vi "test27-MappingRelationshipByLocalRegistration_WithoutSubcriberName.vi"(8 "error in (no error)":errorcluster, 11 "TestCase in":refnum<class "testcase-CSMBroadcast.lvclass">) -> (0 "error out":errorcluster, 3 "TestCase out":refnum<class "testcase-CSMBroadcast.lvclass">)   [LabVIEW 2017, in "testcase-CSMBroadcast.lvclass"]
uses:
  testcase-CSMBroadcast.lvclass
  <vilib>/addons/_JKI Toolkits/VI Tester/TestCase.llb/TestCase.lvclass
  src/user.lib/_NEVSTOP/Communicable State Machine(CSM)/Communicable State Machine.lvlib
  src/user.lib/_NEVSTOP/Communicable State Machine(CSM)/_Shared/CSM Shared.lvlib
  C:/Program Files (x86)/National Instruments/LabVIEW 2017/vi.lib/addons/_JKI Toolkits/VI Tester/TestCase.llb/TestCase.lvclass
panel:
  out "Loop Count":i32
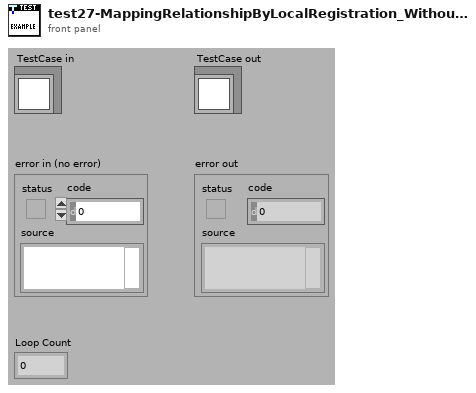
[diagram p1: front panel]
types:
  T1 = cluster{"Status":string, "Source CSM":string, "Target CSM":string, "Target API":string}[]
  T2 = typedef "Communicable State Machine.lvlib/CSM - Broadcast Message Type.ctl" = enum16{"<Null>", "Status", "Interrupt"}
  T3 = cluster{"Status":string, "Source CSM":string, "Target CSM":string, "Target API":string, "Register Type":T2}[]
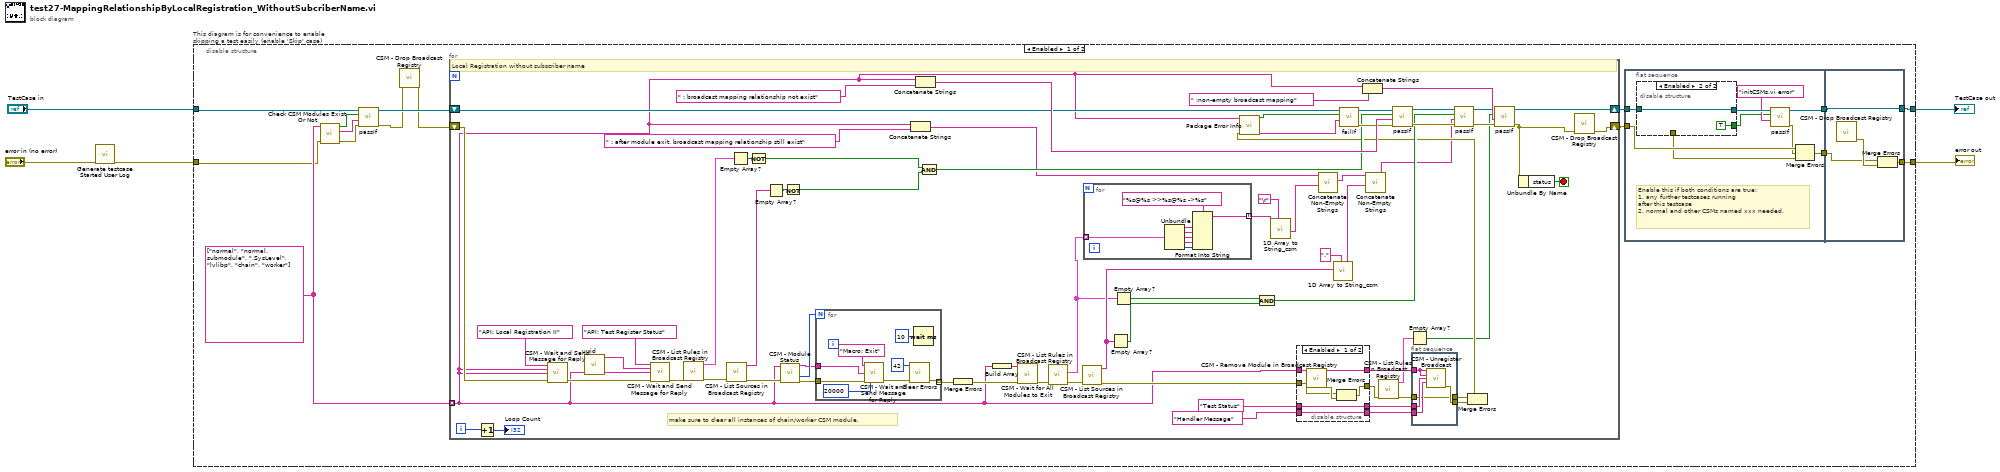
[diagram p0: block diagram]
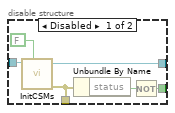
[diagram p2: hidden frame]
diagram:
  n1 = call "Generate testcase Started User Log.vi"("Error In"="error in (no error)") -> ("error out"=w1:errorcluster)  [unwired: 10 in]
  n2 = disable-structure "This diagram is for convenience to enable skipping a test easily (enable 'Skip' case)" shown="Enabled" {
    disable-tunnel: "TestCase in" -> [w16 w147]
    disable-tunnel: [w10 w145] -> w2
    disable-tunnel: [w8 w146] -> w4
    disable-tunnel: w1 -> [w15 w144]
    frame Enabled {
      w17 = string[] ["normal", "normal.submodule", ".SysLevel", "lvlibp", "chain", "worker"]
      n3 = call "Check CSM Modules Exist Or Not.vi"("error in"=w15, "CSM names in"=w17) -> ("error out"=w18:errorcluster, "Debug string"=w19:string, "All Modules Exist?"=w20:bool)  [unwired: 7 in]
      n4 = call-dynamic "passIf.vi"("error in (no error)"=w18, "message (\"\")"=w19, "pass"=w20, "TestCase in"=w16) -> ("error out"=w7:errorcluster, "TestCase out"=w14:refnum<class "testcase-CSMBroadcast.lvclass">)  [unwired: 6 in]
      n5 = call "CSM - Drop Broadcast Registry.vi"("Error In"=w7) -> ("error out"=w6:errorcluster)  [unwired: 14 in]
      n6 = for {
        tunnel: w17 -> [w43] mode=indexing
        shift-right: [w96] -> w11
        shift-left: w14 -> [w83]
        shift-right: [w56] -> w9
        shift-left: w6 -> [w95]
        i -> [w102]
        stop <- w105 stop-if-true
        # "make sure to clear all instances of chain/worker CSM module."
        # "Local Registration without subscriber name"
        n7 = Increment(x=w102) -> (x+1=→"Loop Count":i32)
        n8 = call "CSM - Wait and Send Message for Reply.vi"("State"="API: Local Registration II", "Arguments (\"\")"=w43, "Target Module"=w43, "Error In (No Error)"=w95) -> ("error out"=w110:errorcluster)  [unwired: 8 in, 3 out]
        n9 = call "uuid.vi"() -> ("UUID"=w108:string)  [unwired: 11 in]
        n10 = call "CSM - Wait and Send Message for Reply.vi"("State"="API: Test Register Status", "Arguments (\"\")"=w108, "Target Module"=w43, "Error In (No Error)"=w110) -> ("error out"=w107:errorcluster)  [unwired: 8 in, 3 out]
        n11 = call "CSM - List Rules in Broadcast Registry.vi"("error in (no error)"=w107) -> ("error out"=w104:errorcluster, "Rule Entries"=w100:T1)  [unwired: 8 in, 1 out]
        n12 = call "CSM - List Sources in Broadcast Registry.vi"("error in (no error)"=w104) -> ("error out"=w92:errorcluster, "Broadcast Names"=w97:string[])  [unwired: 9 in]
        n13 = Empty Array?(array=w100) -> (empty?=w99:bool)
        n14 = Not(x=w99) -> (.not. x?=w81:bool)
        n15 = Empty Array?(array=w97) -> (empty?=w98:bool)
        n16 = call "CSM - Module Status.vi"("Error In"=w92, "CSM Name"=w43) -> ("error out"=w91:errorcluster, "#Nodes"=w94:i32, "CSM Name (Dup)"=w93:string)  [unwired: 5 in, 2 out]
        n17 = Not(x=w98) -> (.not. x?=w80:bool)
        n18 = for {
          N: w94 -> [_]
          tunnel: [w139] -> w106 mode=indexing
          tunnel: w93 -> [w142]
          tunnel: w91 -> [w141]
          n19 = call "CSM - Wait and Send Message for Reply.vi"("State"="Macro: Exit", "Target Module"=w142, "Error In (No Error)"=w141, "Response Timeout (-2 Using Global Settings)"=20000 ("Wait (5000ms)")) -> ("error out"=w140:errorcluster)  [unwired: 8 in, 3 out]
          n20 = call <vilib>:"Clear Errors.vi"("error in (no error)"=w140, "specific error code to clear (0: all)"=42) -> ("error out"=w139:errorcluster)  [unwired: 4 in, 1 out]
          n21 = Wait (ms)(milliseconds to wait=u32 10) -> ()  [unwired: 1 out]
        }
        n22 = Concatenate Strings(w43, " : after module exit, broadcast mapping relationship still exist" ("string")) -> (w51:string)
        n23 = Concatenate Strings(w43, " : broadcast mapping relationship not exist" ("string")) -> (w87:string)
        n24 = And(x=w81, y=w80) -> (x .and. y?=w77:bool)
        n25 = Merge Errors(w106) -> (w45:errorcluster)
        n26 = Build Array(w43) -> (w42:string[])
        n27 = call "CSM - Wait for All Modules to Exit.vi"("Error In"=w45, "CSM Names"=w42) -> ("error out"=w44:errorcluster)  [unwired: 7 in, 2 out]
        n28 = call "CSM - List Rules in Broadcast Registry.vi"("error in (no error)"=w44) -> ("error out"=w103:errorcluster, "Rule Entries with Register Type"=w49:T3)  [unwired: 8 in, 1 out]
        n29 = call "CSM - List Sources in Broadcast Registry.vi"("error in (no error)"=w103) -> ("error out"=w63:errorcluster, "Broadcast Names"=w53:string[])  [unwired: 9 in]
        n30 = for {
          tunnel: w49 -> [w119] mode=indexing
          tunnel: [w113] -> w46 mode=indexing
          n31 = Unbundle(w119) -> ("Status"=w118:string, "Source CSM"=w117:string, "Target CSM"=w116:string, "Target API"=w115:string, "Register Type"=w114:T2)
          n32 = Format Into String(format string="%s@%s >>%s@%s ->%s", w118, w117, w116, w115, w114) -> (resulting string=w113:string)  [unwired: 2 in, 1 out]
        }
        n33 = Empty Array?(array=w53) -> (empty?=w78:bool)
        n34 = Empty Array?(array=w49) -> (empty?=w79:bool)
        n35 = And(x=w79, y=w78) -> (x .and. y?=w72:bool)
        n36 = call "1D Array to String_csm.vi"("delimiter (Tab)"="\r", "Array of Strings"=w46) -> ("delimited string"=w48:string)  [unwired: 9 in]
        n37 = disable-structure shown="Enabled" {
          disable-tunnel: w63 -> [w125 w134]
          disable-tunnel: [w129 w134] -> w69
          disable-tunnel: w43 -> [w130 w135]
          disable-tunnel: "Test Status" ("Status") -> [w127 w133]
          disable-tunnel: "Handler Message" ("Response Message (If \"\", Same as Source Message)") -> [w126 w132]
          disable-tunnel: [w128 w135] -> w70
          disable-tunnel: [w127 w133] -> w68
          disable-tunnel: [w126 w132] -> w67
          frame Enabled {
            n38 = call "CSM - Remove Module in Broadcast Registry.vi"("CSM Name"=w130) -> ("CSM Name (Dup)"=w128:string, "error out"=w131:errorcluster)  [unwired: 13 in]
            n39 = Merge Errors(w125, w131) -> (w129:errorcluster)
          }
          frame Disabled {
          }
        }
        n40 = call "Concatenate Non-Empty Strings.vi"("String2"=w48, "String1"=w51) -> ("Result String"=w50:string)  [unwired: 6 in]
        n41 = call "1D Array to String_csm.vi"("delimiter (Tab)"=",", "Array of Strings"=w53) -> ("delimited string"=w54:string)  [unwired: 9 in]
        n42 = Concatenate Strings(w43, " :non-empty broadcast mapping" ("string")) -> (w88:string)
        n43 = call "Concatenate Non-Empty Strings.vi"("String2"=w54, "String1"=w50) -> ("Result String"=w55:string)  [unwired: 6 in]
        n44 = call "CSM - List Rules in Broadcast Registry.vi"("error in (no error)"=w69) -> ("error out"=w65:errorcluster, "Rule Entries"=w59:T1)  [unwired: 8 in, 1 out]
        n45 = Empty Array?(array=w59) -> (empty?=w58:bool)
        n46 = flat-sequence {
          tunnel: w70 -> [w124]
          tunnel: w68 -> [w123]
          tunnel: w67 -> [w122]
          tunnel: [w121] -> w66
          tunnel: w65 -> [w120]
          tunnel: [w120] -> w64
          frame #0 {
            n47 = call "CSM - Unregister Broadcast.vi"("CSM Name(Empty for Broadcast Event)"=w124, "Source CSM Name (* as Default)"=w124, "Trigger"=w123, "API (\"*\" as Default)"=w122) -> ("error out"=w121:errorcluster)  [unwired: 10 in, 1 out]
          }
        }
        n48 = Merge Errors(w64, w66) -> (w62:errorcluster)
        n49 = call "Package Error Info.vi"("error in"=w62, "String in"=w43) -> ("packed error info out"=w86:string, "error status"=w85:bool)  [unwired: 8 in]
        n50 = call-dynamic "failIf.vi"("message (\"\")"=w86, "fail"=w85, "TestCase in"=w83) -> ("error out"=w84:errorcluster, "TestCase out"=w82:refnum<class "testcase-CSMBroadcast.lvclass">)  [unwired: 7 in]
        n51 = call-dynamic "passIf.vi"("error in (no error)"=w84, "message (\"\")"=w87, "pass"=w77, "TestCase in"=w82) -> ("error out"=w74:errorcluster, "TestCase out"=w76:refnum<class "testcase-CSMBroadcast.lvclass">)  [unwired: 6 in]
        n52 = call-dynamic "passIf.vi"("error in (no error)"=w74, "message (\"\")"=w55, "pass"=w72, "TestCase in"=w76) -> ("error out"=w73:errorcluster, "TestCase out"=w75:refnum<class "testcase-CSMBroadcast.lvclass">)  [unwired: 6 in]
        n53 = call-dynamic "passIf.vi"("error in (no error)"=w73, "message (\"\")"=w88, "pass"=w58, "TestCase in"=w75) -> ("error out"=w57:errorcluster, "TestCase out"=w96:refnum<class "testcase-CSMBroadcast.lvclass">)  [unwired: 6 in]
        n54 = Unbundle By Name(w57) -> ("status"=w105:bool)
        n55 = call "CSM - Drop Broadcast Registry.vi"("Error In"=w57) -> ("error out"=w56:errorcluster)  [unwired: 14 in]
      }
      n56 = flat-sequence {
        tunnel: w11 -> [w29]
        tunnel: [w27] -> w13
        tunnel: w9 -> [w25]
        tunnel: [w22] -> w12
        tunnel: w13 -> [w40]
        tunnel: [w40] -> w10
        tunnel: [w39] -> w8
        tunnel: w12 -> [w38]
        frame #0 {
          # "Enable this if both conditions are true:\n1. any further testcases running\nafter this testcase\n2. normal and other CSMs named xxx needed."
          n57 = disable-structure shown="Enabled" {
            disable-tunnel: w29 -> [w35 w37]
            disable-tunnel: [w33 w37] -> w28
            disable-tunnel: [w31 _] -> w23
            disable-tunnel: [w30 TRUE ("pass")] -> w21
            frame Disabled {
              n58 = call "InitCSMs.vi"("Enable building lvlibp?"=FALSE, "testcase-CSMStatus in"=w35) -> ("error out"=w31:errorcluster, "testcase-CSMStatus out"=w33:refnum<class "testcase-CSMBroadcast.lvclass">)  [unwired: 8 in]
              n59 = Unbundle By Name(w31) -> ("status"=w32:bool)
              n60 = Not(x=w32) -> (.not. x?=w30:bool)
            }
            frame Enabled {
            }
          }
          n61 = call-dynamic "passIf.vi"("message (\"\")"="initCSMs.vi error" ("message (\"\")"), "pass"=w21, "TestCase in"=w28) -> ("error out"=w24:errorcluster, "TestCase out"=w27:refnum<class "testcase-CSMBroadcast.lvclass">)  [unwired: 7 in]
          n62 = Merge Errors(w25, w24, w23) -> (w22:errorcluster)
        }
        frame #1 {
          n63 = call "CSM - Drop Broadcast Registry.vi"() -> ("error out"=w41:errorcluster)  [unwired: 15 in]
          n64 = Merge Errors(w38, w41) -> (w39:errorcluster)
        }
      }
    }
    frame Disabled {
      # "skip test result while test is under development"
      n65 = call <vilib>:"skip.vi"("error in (no error)"=w144, "TestCase in"=w147) -> ("error out"=w146:errorcluster, "TestCase out"=w145:refnum<class "testcase-CSMBroadcast.lvclass">)  [unwired: 8 in]
    }
  }
  "error out" <- w4
  "TestCase out" <- w2
